vi "DaemonStatus.vi"(8 "error in (no error)":errorcluster, 11 "queue cluster":T2) -> (0 "error out":errorcluster, 2 "status":T1, 3 "queue cluster out":T2)   [LabVIEW 2014]
uses:
  typedefs/clientStatus.ctl
panel:
  # "\"sent\" is briefly on after tcp transmission,\nand it has little meanong to read it asynchronously.\nEssentially this is for now a placeholder"
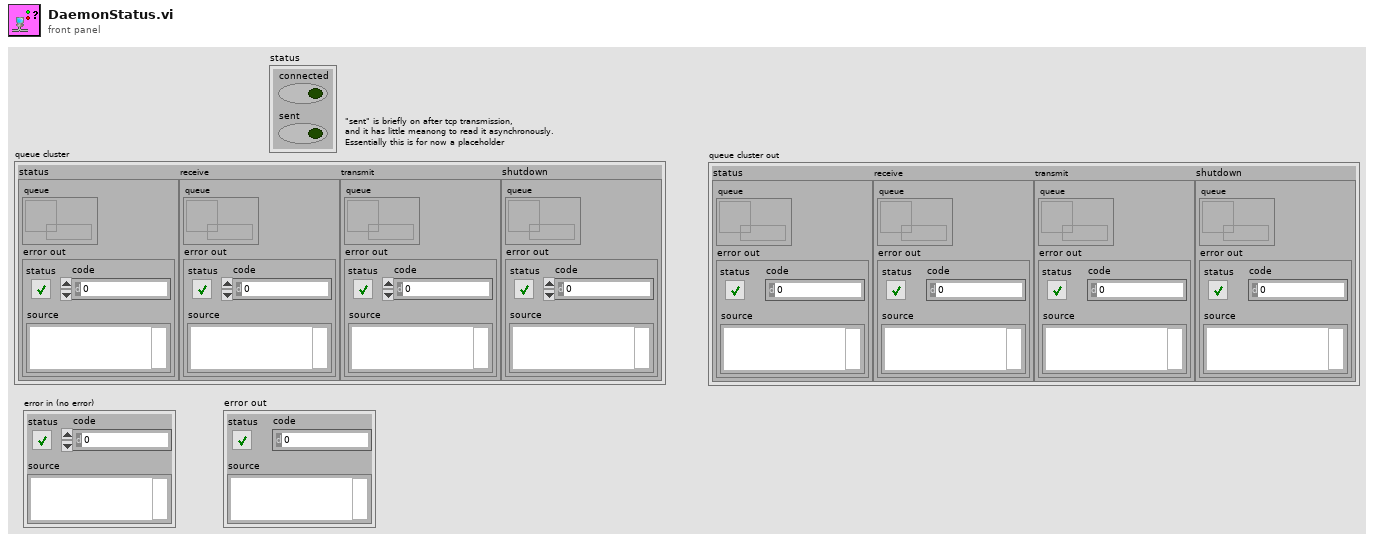
[diagram p1: front panel]
types:
  T1 = typedef "clientStatus.ctl" = cluster{"connected":bool, "sent":bool}
  T2 = cluster{"status":cluster{"queue":refnum<queue>, "error out":errorcluster}, "receive":cluster{"queue":refnum<queue>, "error out":errorcluster}, "transmit":cluster{"queue":refnum<queue>, "error out":errorcluster}, "shutdown":cluster{"queue":refnum<queue>, "error out":errorcluster}}
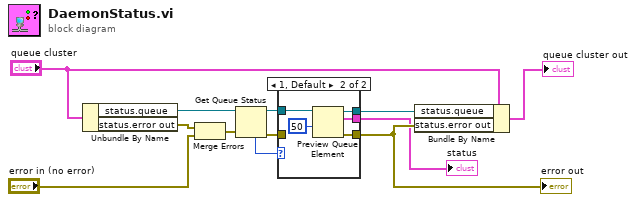
[diagram p0: block diagram]
diagram:
  n1 = Unbundle By Name("queue cluster") -> ("status.queue"=w8:refnum<queue>, "status.error out"=w5:errorcluster)
  n2 = Merge Errors(w5, "error in (no error)") -> (w6:errorcluster)
  n3 = Get Queue Status(queue=w8, error in (no error)=w6) -> (queue out=w7:refnum<queue>, error out=w2:errorcluster, # elements in queue=w3:i32)  [unwired: 1 in, 5 out]
  n4 = case shown="1, Default" w3 {
    tunnel: [w13 w19] -> w10
    tunnel: [w14 w18] -> w9
    tunnel: [_ w15] -> w1
    tunnel: w7 -> [w14 w17]
    tunnel: w2 -> [w13 _]
    frame 0 {
    }
    frame 1, Default {
      n5 = Preview Queue Element(queue=w17, timeout in ms (-1)=50) -> (queue out=w18:refnum<queue>, element=w15:T1, error out=w19:errorcluster)  [unwired: 1 in, 1 out]
    }
  }
  "error out" <- w10
  "status" <- w1
  n6 = Bundle By Name(cluster="queue cluster", "status.queue"=w9, "status.error out"=w10) -> (→"queue cluster out":T2)
